vi "PH_PILS.set Laser Shutters.vi"(0 "i ref in":refnum<vi>, 5 "error in":errorcluster) -> (14 "i ref out":refnum<vi>, 19 "error out":errorcluster)   [LabVIEW 2014, in "PH_PILS.lvlib"]
doc: "This VI calculates and indicatzes the state of the laser safety shutters."
uses:
  PH_PILS.lvlib
  PH_Basics/PH_Common/PH_Common.lvlib
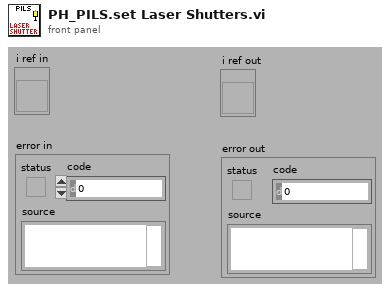
[diagram p1: front panel]
types:
  T1 = typedef "PH_PILS.lvlib/PH_PILS.i attribute.ctl" = cluster{"Boolean":cluster{"GUI Ref":refnum<vi>, "Status":i32}[], "GUI Refs Exp. Shutters":cluster{"1":refnum<vi>, "2":refnum<vi>, "3":refnum<vi>, "4":refnum<vi>}, "Tristate2Run GUI Refs":refnum<vi>[], "EO-Likes":cluster{"GUI Ref":refnum<vi>, "Status":i32}[], "Operation Mode":cluster{"Operation Mode":T2, "GUI":cluster{"Ref State":refnum<vi>, "Ref":refnum<vi>}, "Servicemode":cluster{"Tagname":string, "Status":i32}, "Labormode":cluster{"Tagname":string, "Status":i32}, "Searchmode":cluster{"Tagname":string, "Status":i32}, "Shotmode":cluster{"Tagname":string, "Status":i32}}, "Submode":cluster{"Submode":T3, "GUI":cluster{"Ref State":refnum<vi>, "Ref":refnum<vi>}, "Submode":cluster{"Tagname":string, "Status":i32}}, "Experiment":cluster{"Experiment":enum16{"unknown", "intern", "4 (Z6)", "3", "2", "1"}, "GUI":cluster{"Ref State":refnum<vi>, "Ref":refnum<vi>}, "intern":cluster{"Tagname":string, "Status":i32}, "Exp 4":cluster{"Tagname":string, "Status":i32}, "Exp 3":cluster{"Tagname":string, "Status":i32}, "Exp 2":cluster{"Tagname":string, "Status":i32}, "Exp 1":cluster{"Tagname":string, "Status":i32}}, "TristateNormal":cluster{"GUI Ref":refnum<vi>, "Status":i32}[], "Door Tags":cluster{"GUI Ref":refnum<vi>, "Status":i32}[], "GUIlessTags":cluster{"Name":string, "Status":i32}[], "Beamline GUI Refs":refnum<vi>[], "Special Boolean":cluster{"GUI Ref":refnum<vi>, "Status":i32}[], "Laserpower":cluster{"GUI Ref":refnum<vi>, "Status":i32}[], "Shutter":cluster{"GUI Ref":refnum<vi>, "Status":i32}[], "Tristate EO Like":cluster{"GUI Ref":refnum<vi>, "Status":i32}[], "PP":cluster{"GUI Ref":refnum<vi>, "Status":i32, "Head Ref":refnum<vi>, "Slider Ref":refnum<vi>}[], "Switch Knobs":cluster{"GUI Ref":refnum<vi>, "Status":i32}[], "Latch Knob GUI Refs":refnum<vi>[], "FailureCounter":i32, "Enabled Status":cluster{"Laser":i32, "PreAmp":i32, "MainAmp":i32}, "Mercury":refnum<vi>, "Instance Rods":string, "Logfile":path, "Beckhoff-Instance Internal":string, "Beckhoff-Instance External":string, "Enabling Rights":cluster{"Name":string, "Password":string, "PA?":bool, "MA?":bool, "Exp?":bool}[]}
  T2 = typedef "PH_PILS.lvlib/PH_PILS.Operation Mode.ctl" = enum16{"unknown", "Service", "Labor", "Search", "Shot"}
  T3 = typedef "PH_PILS.lvlib/PH_PILS.Submode.ctl" = enum16{"unknown", "HV-Normal", "HV-Test"}
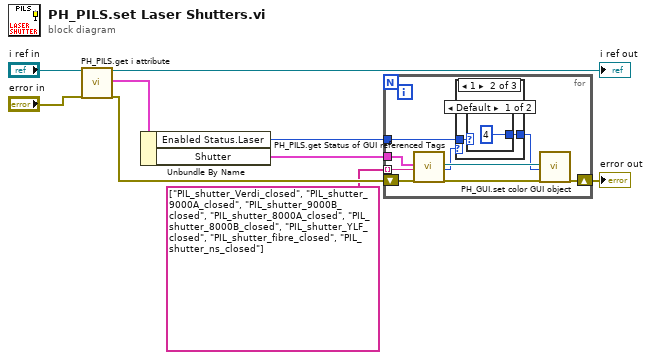
[diagram p0: block diagram]
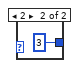
[diagram p3: hidden frame]
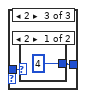
[diagram p4: hidden frame]
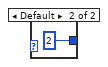
[diagram p5: hidden frame]
diagram:
  n1 = call "PH_PILS.get i attribute.vi"("i ref in"="i ref in", "error in (no error)"="error in") -> ("i ref out"=→"i ref out":refnum<vi>, "i attribute"=w6:T1, "error out"=w4:errorcluster)  [unwired: 15 in]
  n2 = Unbundle By Name(w6) -> ("Enabled Status.Laser"=w1:i32, "Shutter"=w5:cluster{"GUI Ref":refnum<vi>, "Status":i32}[])
  n3 = for {
    tunnel: w5 -> [w18]
    shift-right: [w15] -> w3
    shift-left: w4 -> [w16]
    tunnel: string[] ["PIL_shutter_Verdi_closed", "PIL_shutter_9000A_closed", "PIL_shutter_9000B_closed", "PIL_shutter_8000A_closed", "PIL_shutter_8000B_closed", "PIL_shutter_YLF_closed", "PIL_shutter_fibre_closed", "PIL_shutter_ns_closed"] -> [w13] mode=indexing
    tunnel: w1 -> [w10]
    n4 = call "PH_PILS.get Status of GUI referenced Tags.vi"("Tags"=w18, "Tagname"=w13, "error in"=w16) -> ("GUI Ref"=w14:refnum<vi>, "Status"=w12:i32, "error out"=w17:errorcluster)  [unwired: 13 in, 1 out]
    n5 = case shown="1" w12 {
      selector: w12 -> [w19 _ _]
      tunnel: [w19 w21 w25] -> w11
      tunnel: w10 -> [_ w20 w24]
      frame 0, Default {
      }
      frame 1 {
        n6 = case shown="Default" w20 {
          tunnel: [4 3] -> w21
          frame Default {
          }
          frame 2 {
          }
        }
      }
      frame 2 {
        n7 = case shown="2" w24 {
          tunnel: [4 ("Status") 2 ("Status")] -> w25
          frame 2 {
          }
          frame Default {
          }
        }
      }
    }
    n8 = call "PH_GUI.set color GUI object.vi"("GUI object Ref"=w14, "State"=w11, "error in (no error)"=w17) -> ("error out"=w15:errorcluster)  [unwired: 16 in]
  }
  "error out" <- w3
